vi "Optical Line Measurement.vi"(0 "object distance / mm":dbl caption="g / mm", 1 "image distance / mm":dbl caption="b / mm", 2 "Line Points":T1, 5 "error in (no error)":errorcluster, 8 "Pixel width / mm":dbl=0.003, 10 "Pixel height / mm":dbl=0.003) -> (14 "object / mm":dbl caption="G / mm", 19 "error out":errorcluster)   [LabVIEW 2016, in "MSC Image.lvclass"]
doc: "After the estimation of the image distance, this VI calculates the dimension of an object with known distance marked by Line Points."
uses:
  MSC Image.lvclass
  controls/Contour.ctl
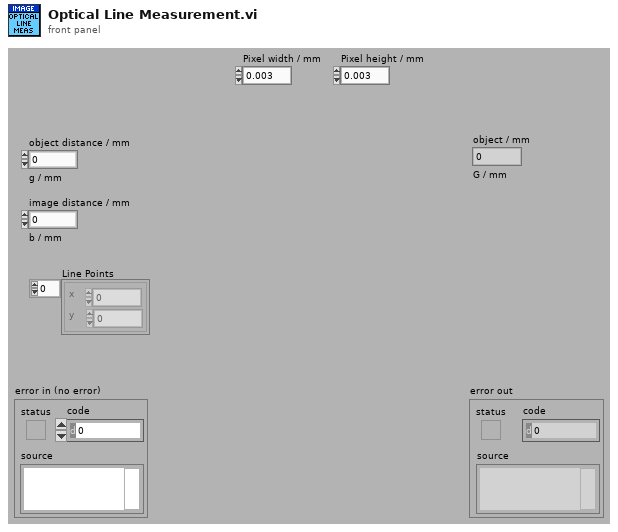
[diagram p1: front panel]
types:
  T1 = typedef "MSC Image.lvclass/Contour.ctl" = cluster{"x":i16, "y":i16}[]
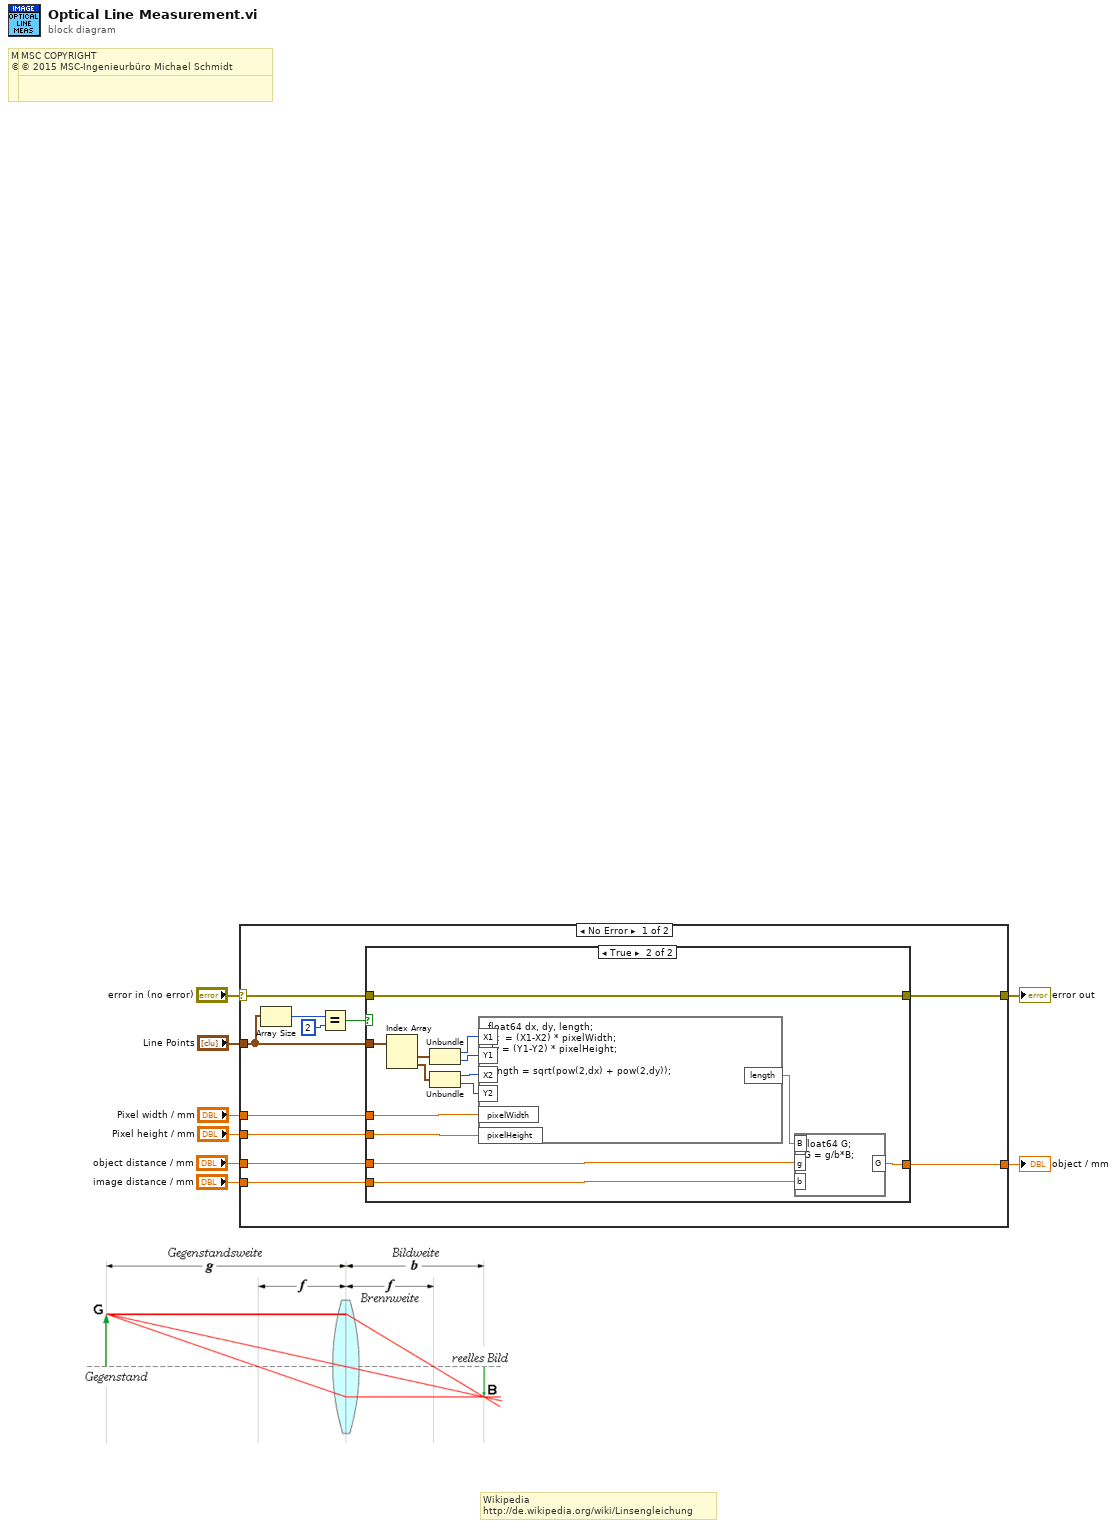
[diagram p0: block diagram]
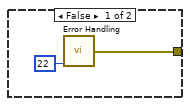
[diagram p2: hidden frame]
diagram:
  # "MSC COPYRIGHT\n© 2016 MSC-Ingenieurbüro Michael Schmidt"
  # "MSC COPYRIGHT\n© 2016 MSC-Ingenieurbüro Michael Schmidt"
  # "MSC COPYRIGHT\n© 2015 MSC-Ingenieurbüro Michael Schmidt"
  # "MSC COPYRIGHT\n© 2015 MSC-Ingenieurbüro Michael Schmidt"
  # "Wikipedia\nhttp://de.wikipedia.org/wiki/Linsengleichung"
  n1 = case shown="No Error" "error in (no error)" {
    selector: "error in (no error)" -> [w19 w36]
    tunnel: [w15 w36] -> w1
    tunnel: "Line Points" -> [w14 _]
    tunnel: "image distance / mm" -> [w13 _]
    tunnel: "object distance / mm" -> [w12 _]
    tunnel: [w11 _] -> w5
    tunnel: "Pixel width / mm" -> [w10 _]
    tunnel: "Pixel height / mm" -> [w9 _]
    frame No Error {
      n2 = Array Size(array=w14) -> (size(s)=w18:i32)
      n3 = Equal?(x=w18, y=2) -> (x = y?=w16:bool)
      n4 = case shown="True" w16 {
        tunnel: w19 -> [_ w25]
        tunnel: [w20 w25] -> w15
        tunnel: w14 -> [_ w35]
        tunnel: w13 -> [_ w23]
        tunnel: w12 -> [_ w22]
        tunnel: [_ w24] -> w11
        tunnel: w10 -> [_ w27]
        tunnel: w9 -> [_ w26]
        frame False {
          n5 = call "Error Handling.vi"("return type"=22) -> ("error out"=w20:errorcluster)  [unwired: 13 in, 1 out]
        }
        frame True {
          n6 = Index Array(array=w35) -> (element #1=w34:cluster{"x":i16, "y":i16}, element #2=w33:cluster{"x":i16, "y":i16})  [unwired: 2 in]
          n7 = Unbundle(w34) -> ("x"=w31:i16, "y"=w30:i16)
          n8 = Unbundle(w33) -> ("x"=w29:i16, "y"=w28:i16)
          n9 = formula code="float64 dx, dy, length;\ndx  = (X1-X2) * pixelWidth;\ndy = (Y1-Y2) * pixelHeight;\n\nlength = sqrt(pow(2,dx) + pow(2,dy));"("X1"=w31, "Y1"=w30, "X2"=w29, "Y2"=w28, "pixelWidth"=w27, "pixelHeight"=w26) -> ("length"=w32:dbl)
          n10 = formula code="float64 G;\nG = g/b*B;"("B"=w32, "g"=w22, "b"=w23) -> ("G"=w24:dbl)
        }
      }
    }
    frame Error {
    }
  }
  "error out" <- w1
  "object / mm" <- w5
